vi "GFITS_header_operate.vi"(10 "expression":string, 11 "Database RefNum in":T1) -> (2 "value":string, 3 "numeric data type":i32)   [LabVIEW 2016]
uses:
  DBSHAND/private/vis/DatabaseHand_RefNum.ctl
  DBSHAND/private/vis/DatabaseHand_Element_Get(string).vi
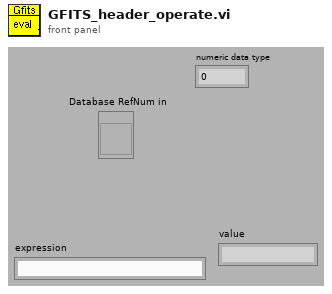
[diagram p1: front panel]
types:
  T1 = typedef "DatabaseHand_RefNum.ctl" = refnum<vi>
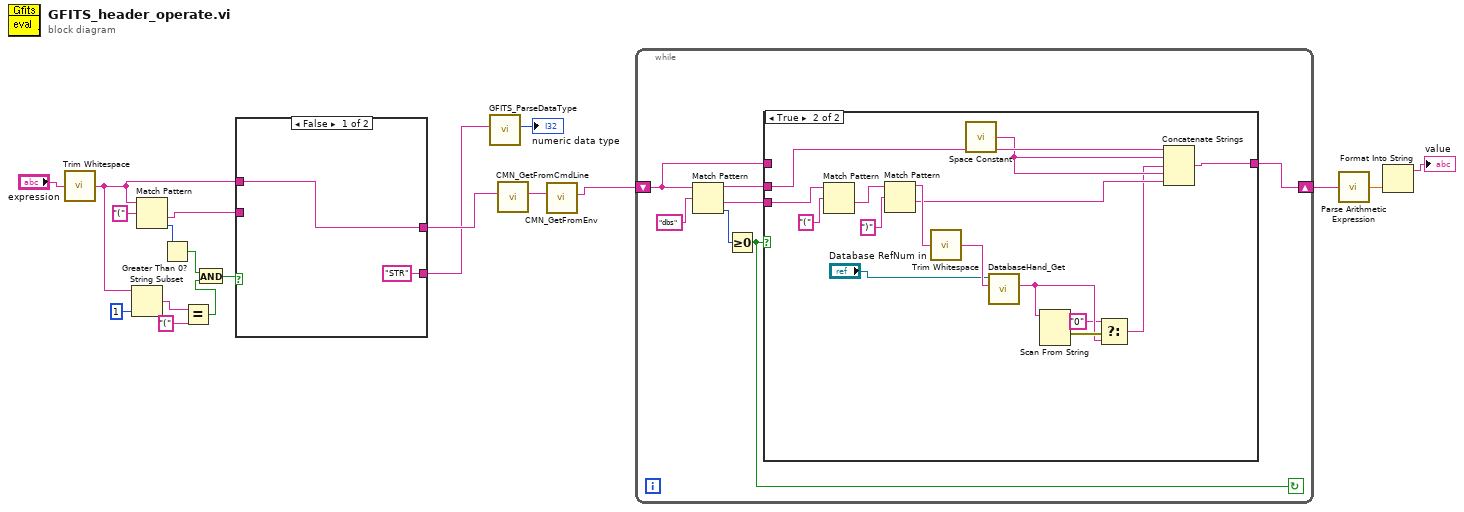
[diagram p0: block diagram]
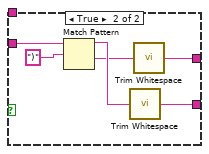
[diagram p2: hidden frame]
diagram:
  n1 = call <vilib>:"Trim Whitespace.vi"("string"="expression") -> ("trimmed string"=w1:string)  [unwired: 1 in]
  n2 = String Subset(string=w1, length (rest)=1 ("length (rest)")) -> (substring=w8:string)  [unwired: 1 out]
  n3 = Match Pattern(string=w1, regular expression="(") -> (after substring=w4:string, offset past match=w12:i32)  [unwired: 3 out]
  n4 = Greater Than 0?(x=w12) -> (x > 0?=w11:bool)
  n5 = Equal?(x=w8, y="(") -> (x = y?=w9:bool)
  n6 = And(x=w11, y=w9) -> (x .and. y?=w5:bool)
  n7 = case shown="False" w5 {
    tunnel: w4 -> [_ w26]
    tunnel: [w20 w23] -> w3
    tunnel: ["STR" ("trimmed string") w22] -> w2
    tunnel: w1 -> [w20 _]
    frame False {
    }
    frame True {
      n8 = Match Pattern(string=w26, regular expression=")") -> (before substring=w25:string, after substring=w24:string)  [unwired: 3 out]
      n9 = call <vilib>:"Trim Whitespace.vi"("string"=w25) -> ("trimmed string"=w22:string)  [unwired: 1 in]
      n10 = call <vilib>:"Trim Whitespace.vi"("string"=w24) -> ("trimmed string"=w23:string)  [unwired: 1 in]
    }
  }
  n11 = call "GFITS_ParseDataType.vi"("string type"=w2) -> ("numeric type"=→"numeric data type":i32)  [unwired: 10 out]
  n12 = call "CMN_GetFromCmdLine.vi"("str in"=w3) -> ("str out"=w19:string)  [unwired: 10 out]
  n13 = call "CMN_GetFromEnv.vi"("str in"=w19) -> ("str out"=w17:string)  [unwired: 10 out]
  n14 = while {
    shift-right: [w29] -> w16
    shift-left: w17 -> [w31]
    stop <- w30 continue-if-true
    n15 = Match Pattern(string=w31, regular expression="dbs") -> (before substring=w28:string, after substring=w33:string, offset past match=w32:i32)  [unwired: 2 out]
    n16 = Greater Or Equal To 0?(x=w32) -> (x >= 0?=w30:bool)
    n17 = case shown="True" w30 {
      tunnel: w33 -> [_ w49]
      tunnel: w31 -> [w35 _]
      tunnel: [w35 w40] -> w29
      tunnel: w28 -> [_ w43]
      frame False {
      }
      frame True {
        n18 = Match Pattern(string=w49, regular expression="(") -> (after substring=w48:string)  [unwired: 4 out]
        n19 = Match Pattern(string=w48, regular expression=")") -> (before substring=w46:string, after substring=w41:string)  [unwired: 3 out]
        n20 = call <vilib>:"Trim Whitespace.vi"("string"=w46) -> ("trimmed string"=w45:string)  [unwired: 1 in]
        n21 = call <vilib>:"Space Constant.vi"() -> ("String"=w42:string)
        n22 = call-poly "DatabaseHand_Get.vi"("name"=w45, "Database RefNum in"="Database RefNum in") -> ("value"=w38:string)  [unwired: 3 in, 6 out]
        n23 = Scan From String(input string=w38) -> (error out=w39:errorcluster)  [unwired: 3 in, 4 out]
        n24 = Select(t="0", s=w39, f=w38) -> (s? t:f=w36:string)
        n25 = Concatenate Strings(w43, w42, w36, w42, w41) -> (w40:string)
      }
    }
  }
  n26 = call "Parse Arithmetic Expression.vi"("Arithmetic Expression"=w16) -> ("Result"=w15:dbl)
  n27 = Format Into String(w15) -> (resulting string=→"value":string)  [unwired: 3 in, 1 out]
